vi "TextIcon-old.vi"(7 "picture":picture, 9 "rect":T1={"left"=2, "top"=17, "right"=32, "bottom"=32}, 10 "Text 2":string, 11 "Text":u32(colorbox)=6589059) -> (3 ">> TextIcon >>":T2 caption="用户图层")   [LabVIEW 2013]
uses:
  <vilib>/picture/picture.llb/imagedata.ctl
  <vilib>/Utility/miscctls.llb/LVPoint32TypeDef.ctl
  <vilib>/LabVIEW Icon API/API_User Layer Data.ctl
  <vilib>/LabVIEW Icon API/LabVIEW Icon API.lvlib
panel:
  out "array":string[](array[string])
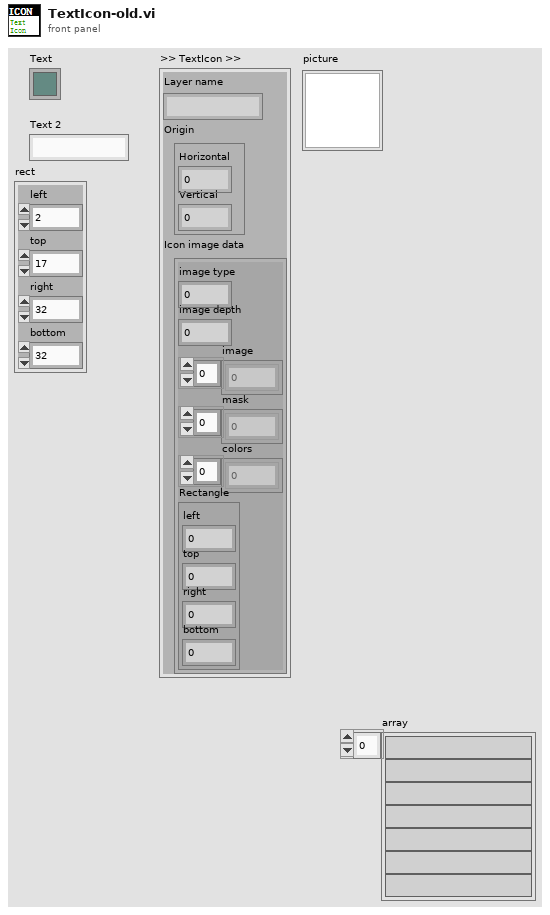
[diagram p1: front panel]
types:
  T1 = cluster{"left":i16, "top":i16, "right":i16, "bottom":i16}
  T2 = typedef "LabVIEW Icon API.lvlib/API_User Layer Data.ctl" = cluster{"Layer name":string, "Origin":T3, "Icon image data":T4}
  T3 = typedef "LVPoint32TypeDef.ctl" = cluster{"Horizontal":i32, "Vertical":i32}
  T4 = typedef "imagedata.ctl" = cluster{"image type":i32, "image depth":i32, "image":u8[], "mask":u8[], "colors":u32[], "Rectangle":cluster{"left":i16, "top":i16, "right":i16, "bottom":i16}}
  T5 = cluster{"Font Name:":string, "Size":i16, "Strikeout?":bool, "Italic?":bool, "Underline?":bool, "Outline?":bool, "Shadow?":bool, "Bold?":bool}
  T6 = enum16{"User-specified Font", "Application Font", "System Font", "Dialog Font"}
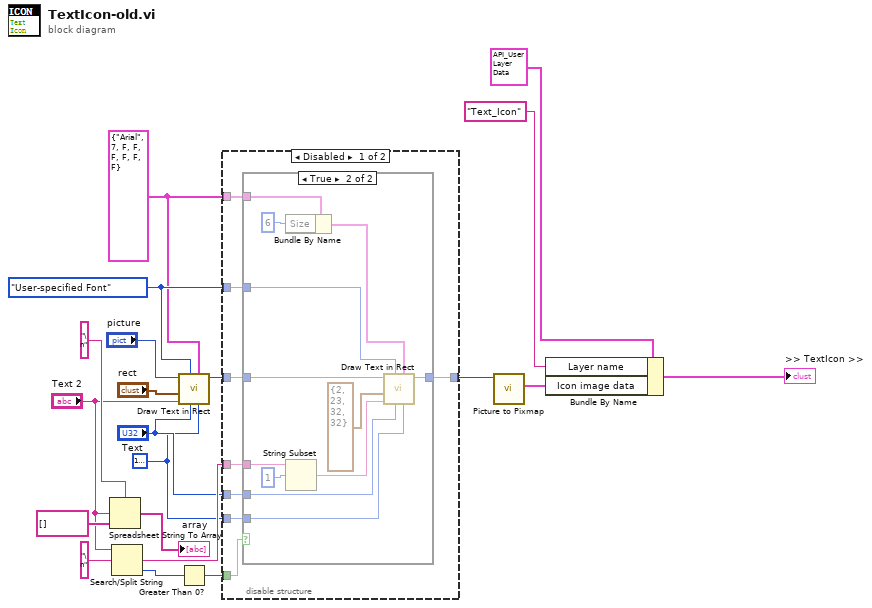
[diagram p0: block diagram]
diagram:
  w6 = T5 {"Font Name:"="Arial", "Size"=7, "Strikeout?"=FALSE, "Italic?"=FALSE, "Underline?"=FALSE, "Outline?"=FALSE, "Shadow?"=FALSE, "Bold?"=FALSE} ("[user-specified font]")
  w7 = T6."User-specified Font" ("desired font(Application)")
  w8 = u32 16777216 ("BG color(transparent)")
  n1 = Spreadsheet String To Array(delimiter (Tab)="\n", spreadsheet string="Text 2", array type (2D Dbl)=string[] []) -> (array=→"array":string[])  [unwired: 1 in]
  n2 = Search/Split String(string="Text 2", search string/char (-)="\n" ("搜索字符串/字符(-)")) -> (match + rest of string=w10:string, offset of match=w15:i32)  [unwired: 1 in, 1 out]
  n3 = call <vilib>:"Draw Text in Rect.vi"("BG color(transparent)"=w8, "[user-specified font]"=w6, "text color(black)"="Text", "desired font(Application)"=w7, "text"="Text 2", "rect"="rect", "picture"="picture") -> ("new picture"=w13:picture)  [unwired: 4 in]
  n4 = Greater Than 0?(x=w15) -> (x > 0?=w11:bool)
  n5 = disable-structure shown="Disabled" {
    disable-tunnel: w13 -> [w28 w42]
    disable-tunnel: [w27 w42] -> w12
    disable-tunnel: w11 -> [w26 _]
    disable-tunnel: w10 -> [w25 _]
    disable-tunnel: "Text" -> [w24 _]
    disable-tunnel: w8 -> [w23 _]
    disable-tunnel: w7 -> [w22 _]
    disable-tunnel: w6 -> [w21 _]
    frame Disabled {
      n6 = case shown="True" w26 {
        tunnel: w28 -> [w29 w41]
        tunnel: [w29 w40] -> w27
        tunnel: w25 -> [_ w38]
        tunnel: w24 -> [_ w35]
        tunnel: w23 -> [_ w34]
        tunnel: w22 -> [_ w33]
        tunnel: w21 -> [_ w32]
        frame False {
        }
        frame True {
          n7 = Bundle By Name(cluster=w32, "Size"=i16 6) -> (w31:T5)
          n8 = String Subset(string=w38, offset (0)=1 ("偏移量(0)")) -> (substring=w37:string)  [unwired: 1 in]
          n9 = call <vilib>:"Draw Text in Rect.vi"("BG color(transparent)"=w34, "[user-specified font]"=w31, "text color(black)"=w35, "desired font(Application)"=w33, "text"=w37, "rect"=T1 {"left"=2, "top"=23, "right"=32, "bottom"=32}, "picture"=w41) -> ("new picture"=w40:picture)  [unwired: 4 in]
        }
      }
    }
    frame Enabled {
    }
  }
  n10 = call <vilib>:"Picture to Pixmap.vi"("picture"=w12) -> ("image data"=w19:T4)  [unwired: 9 in, 1 out]
  n11 = Bundle By Name(cluster=T2 {"Layer name"="", "Origin"={"Horizontal"=0, "Vertical"=0}, "Icon image data"={"image type"=0, "image depth"=0, "image"=[], "mask"=[], "colors"=[], "Rectangle"={"left"=0, "top"=0, "right"=0, "bottom"=0}}} ("User layer"), "Layer name"="Text_Icon", "Icon image data"=w19) -> (→">> TextIcon >>":T2)
